vi "CHD_SIM_Gyro_Open.vi"(11 "Analog Channel":T1=enum."AI 1") -> (0 "error out":errorcluster, 3 "GyroDevRef":T2 {"Sample Rate" min=0.25 max=100.0 step=0.25})   [LabVIEW 2019]
uses:
  <vilib>/Rock Robotics/WPI/Gyro/WPI_GyroDevRef.ctl
  <vilib>/Rock Robotics/SystemInterfaces/AI/FPGA_AIChannel.ctl
  <vilib>/Rock Robotics/SystemInterfaces/spilib/spi_bus.ctl
  <vilib>/Rock Robotics/SystemInterfaces/AI/FPGA_AIGyroChannel.ctl
  CHS_SIM_SIM_Globals.vi
panel:
  # "Analog"
  # "XRS"
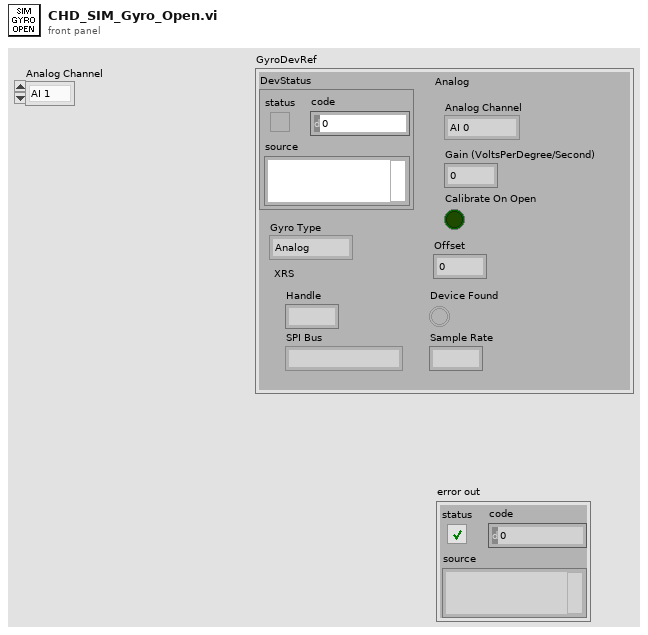
[diagram p1: front panel]
types:
  T1 = typedef "FPGA_AIGyroChannel.ctl" = enum8{"AI 0", "AI 1", "Invalid"}
  T2 = typedef "WPI_GyroDevRef.ctl" = cluster{"DevStatus":errorcluster, "Analog Channel":T3, "Gain (VoltsPerDegree/Second)":dbl, "Gyro Type":enum16{"Analog", "XRS450"}, "Handle":i32, "SPI Bus":T4, "Device Found":bool, "Sample Rate":dbl, "Calibrate On Open":bool, "Offset":dbl}
  T3 = typedef "FPGA_AIChannel.ctl" = enum8{"AI 0", "AI 1", "AI 2", "AI 3", "AI MXP 0", "AI MXP 1", "AI MXP 2", "AI MXP 3", "Invalid"}
  T4 = typedef "spi_bus.ctl" = enum16{"SPI On-Board, CS0", "SPI On-Board, CS1", "SPI On-Board, CS2", "SPI On-Board, CS3", "SPI MXP", "Invalid"}
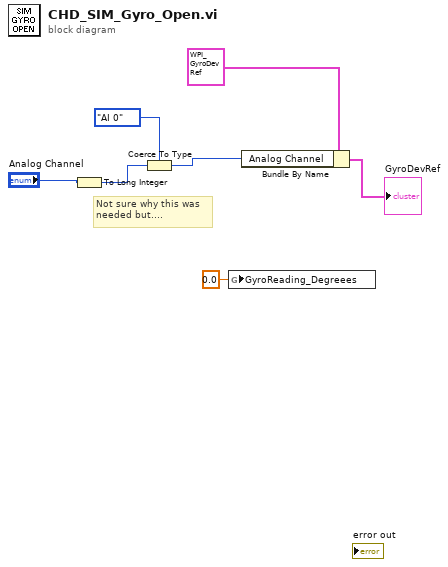
[diagram p0: block diagram]
diagram:
  # "Not sure why this was\nneeded but...."
  n1 = To Long Integer(number="Analog Channel") -> (32bit integer=w2:i32)
  n2 = Coerce To Type(0:w2, 1:FPGA_AIChannel."AI 0" ("Analog Channel")) -> (2:w1:T3)
  n3 = global write "CHS_SIM_SIM_Globals.vi" "GyroReading_Degreees"(0.0 ("GyroReading_Degreees")) -> ()
  n4 = Bundle By Name(cluster=T2 {"DevStatus"={"status"=FALSE, "code"=0, "source"=""}, "Analog Channel"=enum."AI 0", "Gain (VoltsPerDegree/Second)"=0.0, "Gyro Type"=enum."Analog", "Handle"=0, "SPI Bus"=enum."SPI On-Board, CS0", "Device Found"=FALSE, "Sample Rate"=0.0, "Calibrate On Open"=FALSE, "Offset"=0.0} ("GyroDevRef"), "Analog Channel"=w1) -> (→"GyroDevRef":T2)
